vi "test_read_memory.vi"() -> ()   [LabVIEW 2018]
uses:
  <vilib>/rvi/Emulation/niFpgaSctlEmulationGetInTimedLoop.vi
  <vilib>/rvi/Memory/Memory_Emulation/nirvimemoryFastEmulation.vi
  <vilib>/rvi/Memory/Memory_Emulation/nirvimemoryEmulation.vi
  <vilib>/rvi/Emulation/niFpgaEmulationIsFPGAContextNoSignature.vi
  <vilib>/rvi/DataTransferAndStorage/Container/Common/niFpgaContainerGetUniqueNameForEmu.vi
  <vilib>/rvi/Emulation/niFpgaProcessEmulError.vi
  <vilib>/rvi/errors/nirviReportUnexpectedCaseInternalError (U32).vi
  <vilib>/rvi/DataTransferAndStorage/Container/XNode/niFpgaContainer.xnode
panel:
  out "values":dbl[](array[numeric])
  out "Index":u32[](array[numeric])
  out "Waveform Graph 2":dbl[][](graph)
  out "Waveform Graph":dbl[][](graph)
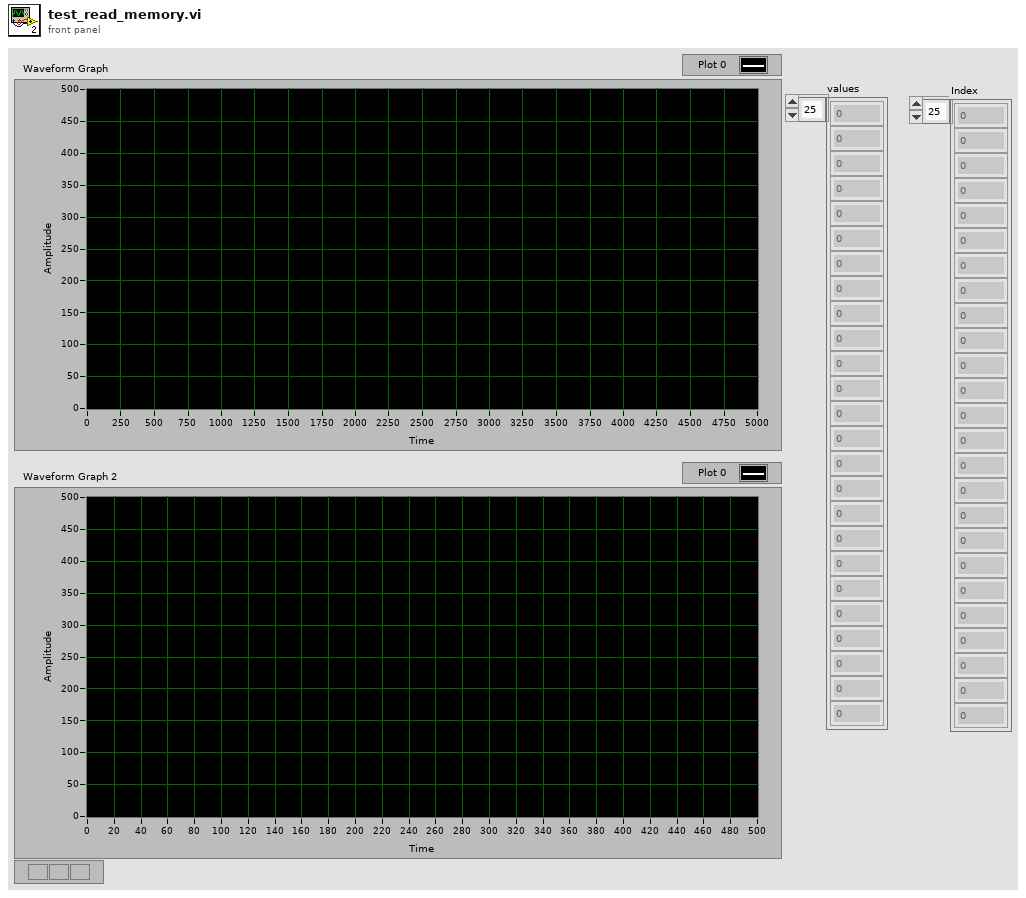
[diagram p1: front panel]
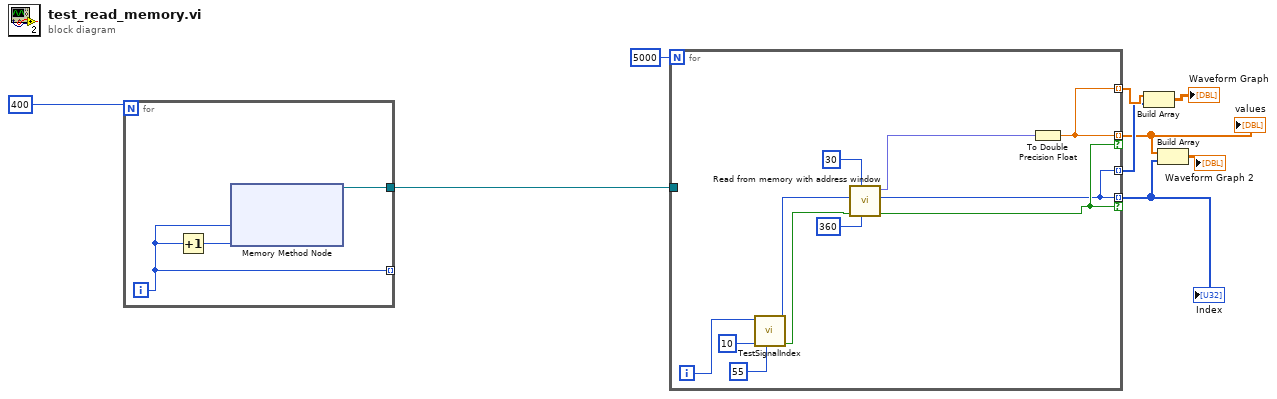
[diagram p0: block diagram]
diagram:
  n1 = for {
    N: 400 -> [_]
    tunnel: [w11] -> _ mode=indexing
    tunnel: [w10] -> w8
    i -> [w11]
    n2 = Increment(x=w11) -> (x+1=w12:i32)
    n3 = xnode ("Memory Method Node")("Address"=w11, "Data"=w12) -> ("Memory Out"=w10:refnum<k21>)  [unwired: 1 in]
  }
  n4 = for {
    N: 5000 -> [_]
    tunnel: w8 -> [_]
    tunnel: [w13] -> w2 mode=indexing if=w15
    tunnel: [w14] -> w3 mode=indexing if=w15
    tunnel: [w14] -> w6 mode=indexing
    tunnel: [w13] -> w5 mode=indexing
    i -> [w21]
    n5 = call "TestSignalIndex.vi"("initial delay"=55, "cycles per sample"=10 ("y"), "index"=w21) -> ("valid out"=w18:bool, "array index"=w17:i32)  [unwired: 7 in]
    n6 = call "Read from memory with address window.vi"("last adress"=u32 360, "First adress"=u32 30, "input valid"=w18, "Address"=w17) -> ("output valid"=w15:bool, "Address out"=w13:u32, "Value out"=w16:fxp<+/-,32,14>)  [unwired: 5 in]
    n7 = To Double Precision Float(number=w16) -> (double precision float=w14:dbl)
  }
  "Index" <- w2
  "values" <- w3
  n8 = Build Array(w6, w5) -> (→"Waveform Graph":dbl[][])
  n9 = Build Array(w3, w2) -> (→"Waveform Graph 2":dbl[][])
